vi "RP read file.vi"(8 "Error In":errorcluster) -> (0 "Error Out":errorcluster)   [LabVIEW 2015]
uses:
  <vilib>/Waveform/WDTOps.llb/WDT Number of Waveform Samples DBL.vi
  <vilib>/measure/NI_MABase.lvlib
panel:
  in  "Pipeline delay":dbl
  out "Frequency":dbl format="%#_6p"
  out "Phase":u32
  out "Frequency word":u32
  out "Waveform Graph":waveform(dbl)[](graph)
  out "group/channel names":string[][](array[string])
  in  "File Path Control":path
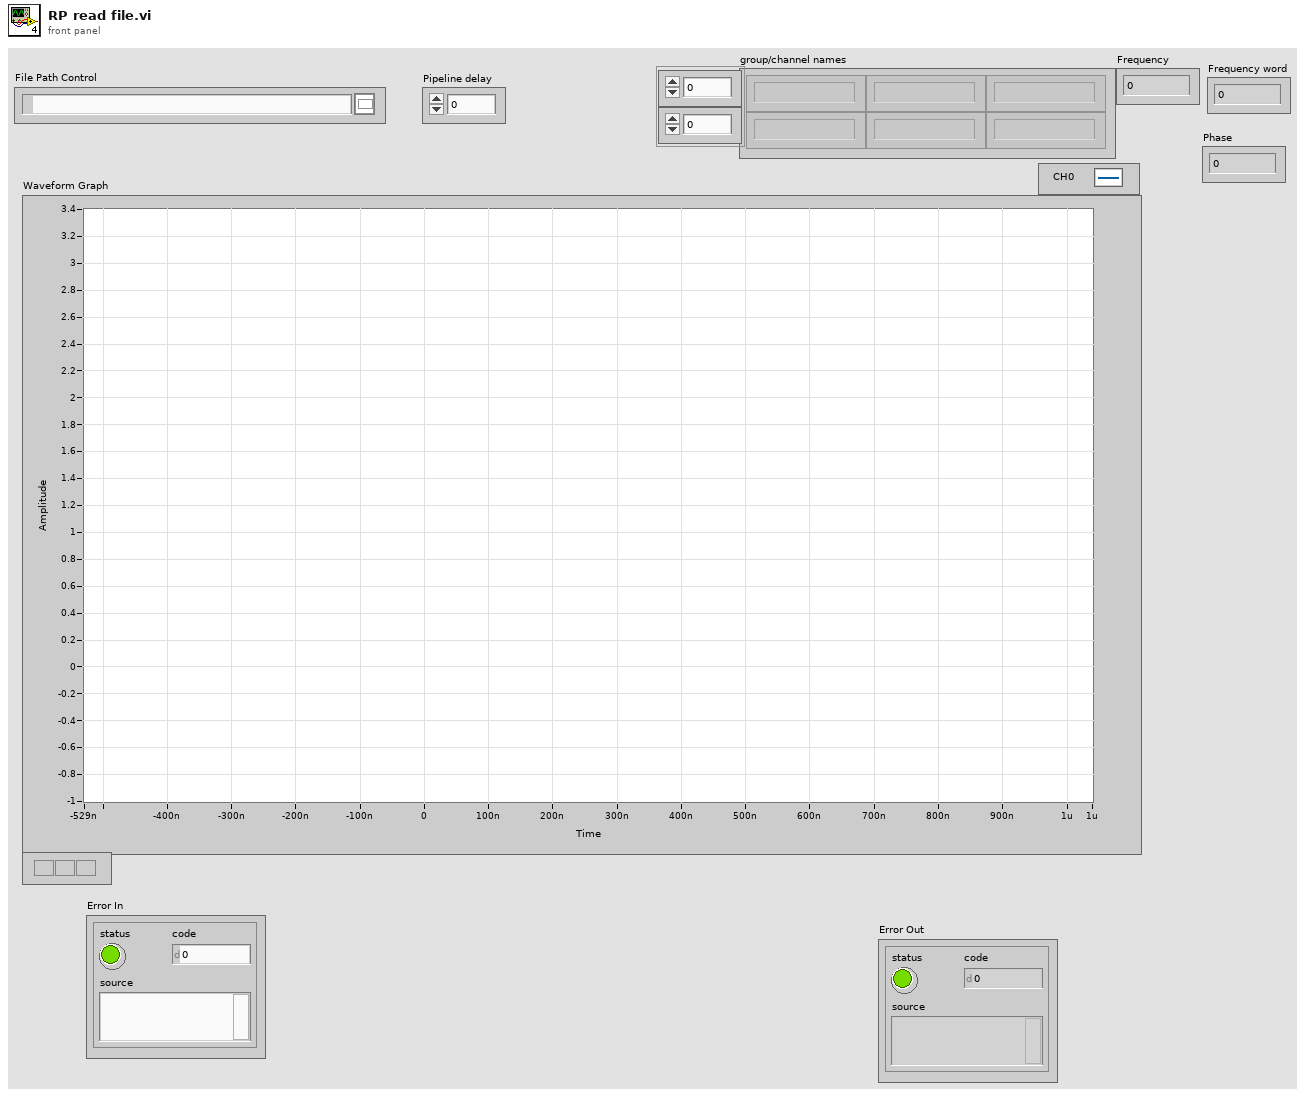
[diagram p1: front panel]
types:
  T1 = enum16{"open", "open or create", "create or replace", "create", "open (read-only)"}
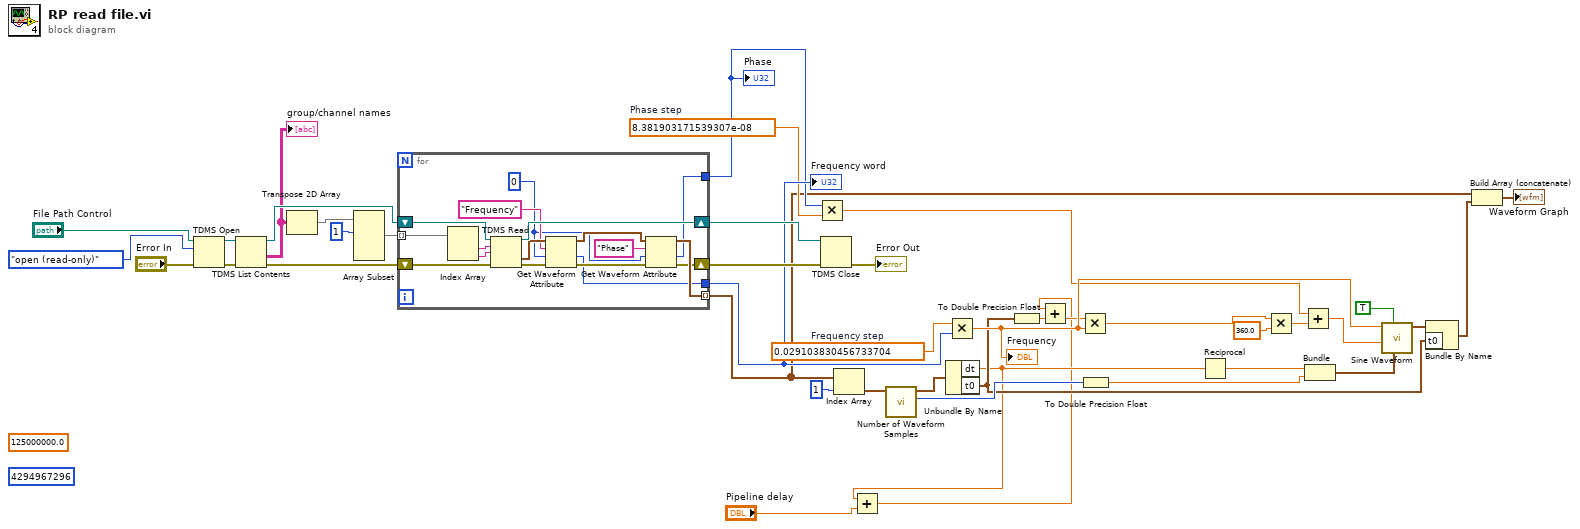
[diagram p0: block diagram]
diagram:
  w22 = 8.381903171539307e-08  # Phase step
  w25 = 0.029103830456733704  # Frequency step
  (unwired) u64 4294967296
  (unwired) 125000000.0
  n1 = TDMS Open(8:"Error In", 10:T1."open (read-only)" ("operation (0:open)"), 11:"File Path Control") -> (0:w39:errorcluster, 3:w38:refnum<k34>)  [unwired: 4 in]
  n2 = TDMS List Contents(4:w39, 7:w38) -> (0:w37:errorcluster, 1:w35:string[][], 3:w36:refnum<k34>)  [unwired: 1 in, 1 out]
  "group/channel names" <- w35
  n3 = Transpose 2D Array(2D array=w35) -> (transposed array=w30:string[][])
  n4 = Array Subset(array=w30, index (row)=1 ("index")) -> (w31:string[][])  [unwired: 3 in]
  n5 = for {
    shift-right: [w47] -> w33
    shift-left: w37 -> [w59]
    shift-right: [w54] -> w34
    shift-left: w36 -> [w58]
    tunnel: w31 -> [w57] mode=indexing
    tunnel: [w49] -> w7 mode=indexing
    tunnel: [w44] -> w24
    tunnel: [w43] -> w23
    w45 = u32 0 ("index")
    n6 = Index Array(array=w57) -> (element #1=w55:string, element #2=w56:string)  [unwired: 2 in]
    n7 = TDMS Read(0:w58, 5:w55, 7:w56, 11:w59) -> (4:w54:refnum<k34>, 10:w53:waveform(dbl), 15:w51:errorcluster)  [unwired: 4 in, 3 out]
    n8 = Get Waveform Attribute(4:w51, 5:w45, 6:"Frequency" ("name"), 7:w53) -> (0:w48:errorcluster, 1:w44:u32, 3:w50:waveform(dbl))  [unwired: 1 out]
    n9 = Get Waveform Attribute(4:w48, 5:w45, 6:"Phase" ("name"), 7:w50) -> (0:w47:errorcluster, 1:w43:u32, 3:w49:waveform(dbl))  [unwired: 1 out]
  }
  "Frequency word" <- w24
  "Phase" <- w23
  n10 = Multiply(x=w23, y=w22) -> (x*y=w12:dbl)
  n11 = TDMS Close(8:w33, 11:w34) -> (0:→"Error Out":errorcluster)  [unwired: 1 out]
  n12 = Index Array(array=w7, index=1) -> (element=w27:waveform(dbl))
  n13 = call-poly <vilib>:"Number of Waveform Samples.vi"("waveform in"=w27) -> ("number of samples"=w21:i32, "waveform out"=w26:waveform(dbl))  [unwired: 8 in, 1 out]
  n14 = Unbundle By Name(w26) -> ("dt"=w3:dbl, "t0"=w8:timestamp)
  n15 = Add(x=w3, y="Pipeline delay") -> (x+y=w1:dbl)
  n16 = Multiply(x=w25, y=w24) -> (x*y=w16:dbl)
  "Frequency" <- w16
  n17 = To Double Precision Float(number=w8) -> (double precision float=w15:dbl)
  n18 = Add(x=w1, y=w15) -> (x+y=w2:dbl)
  n19 = Multiply(x=w2, y=w16) -> (x*y=w14:dbl)
  n20 = To Double Precision Float(number=w21) -> (double precision float=w19:dbl)
  n21 = Reciprocal(x=w3) -> (1/x=w20:dbl)
  n22 = Multiply(x=w14, y=360.0) -> (x*y=w11:dbl)
  n23 = Add(x=w12, y=w11) -> (x+y=w10:dbl)
  n24 = Bundle(w20, w19) -> (w18:cluster{dbl, dbl})  [unwired: 1 in]
  n25 = call <vilib>:"Sine Waveform.vi"("sampling info"=w18, "reset signal"=TRUE, "phase"=w10, "frequency"=w16) -> ("signal out"=w9:waveform(dbl))  [unwired: 6 in, 1 out]
  n26 = Bundle By Name(cluster=w9, "t0"=w8) -> (w6:waveform(dbl))
  n27 = Build Array (concatenate)(w7, w6) -> (→"Waveform Graph":waveform(dbl)[])
